vi "Initialize-values.vi"(8 "error in":errorcluster, 11 "UI ref. in":refnum<data-value>) -> (0 "error IO":errorcluster, 3 "UI ref.":refnum<data-value>)   [LabVIEW 2013, in "CameraVision.lvlib" / "CV-UI.lvclass"]
doc: "This function resets the values of the GUI buttons and selectors to consistent defaults.\nThe purpose is to present a consistent GUI after an unexpected program shutdown."
uses:
  CV-UI.lvclass
  CV-UI.lvclass/CV-UI.ctl
  Camera-selector.ctl
  Image-selector.ctl
  Main/Mapping/Mapping-characteristic.ctl
  Settings-source.ctl
  Read Control refs.vi
  Main/Mapping/CV-Mapping.lvclass
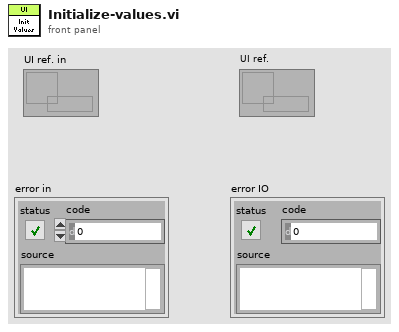
[diagram p1: front panel]
types:
  T1 = typedef "CameraVision.lvlib/CV-UI.lvclass/Camera-selector.ctl" = enum16{"Camera 1", "Camera 2"}
  T2 = typedef "CameraVision.lvlib/CV-UI.lvclass/Image-selector.ctl" = enum16{"Original", "Corrected", "Binary"}
  T3 = typedef "CameraVision.lvlib/CV-Mapping.lvclass/Mapping-characteristic.ctl" = enum16{"Average intensity [0-255]", "Peak intensity [0-255]", "Melt-pool size [mm²]", "Melt-pool aspect ratio []", "Melt-pool fragments []", "Average temperature [°C]", "Max. temperature [°C]", "Min. temperature [°C]", "Std. dev. temperature [°C]"}
  T4 = typedef "CameraVision.lvlib/CV-UI.lvclass/Settings-source.ctl" = enum16{"Custom", "Default", "Last used", "File"}
  T5 = typedef "CameraVision.lvlib/CV-UI.lvclass/Control-names.ctl" = enum16{"Start acquisition", "Activate", "Stop acquisition", "Settings type", "Load settings", "Save settings", "Import images", "Camera selector", "Image type selector", "Batch browser", "Image refresh", "Parameter tabs", "Displays", "Processing tabs", "Processing selector", "Map characteristic", "Show info", "Manual trigger"}
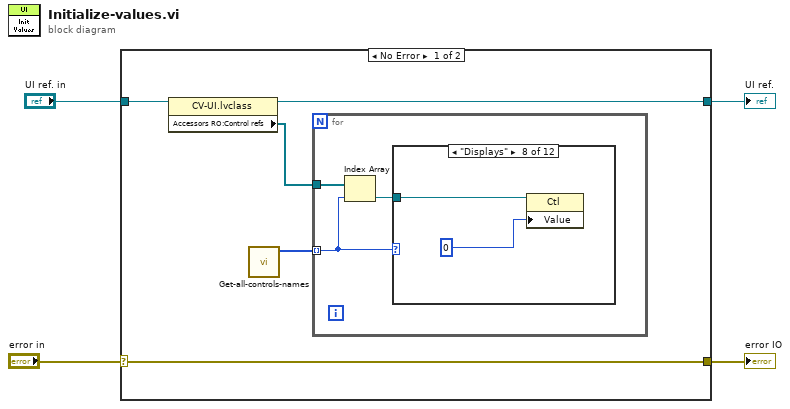
[diagram p0: block diagram]
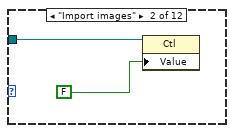
[diagram p3: hidden frame]
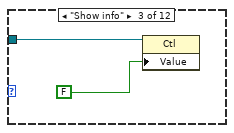
[diagram p4: hidden frame]
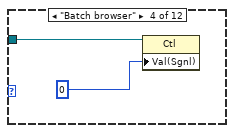
[diagram p5: hidden frame]
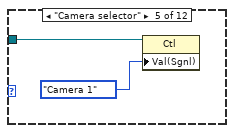
[diagram p6: hidden frame]
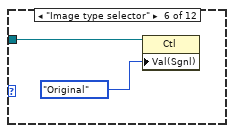
[diagram p7: hidden frame]
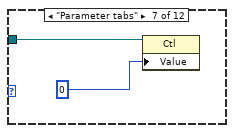
[diagram p8: hidden frame]
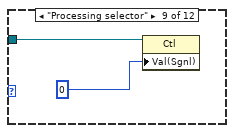
[diagram p9: hidden frame]
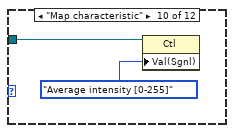
[diagram p10: hidden frame]
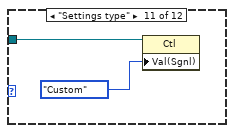
[diagram p11: hidden frame]
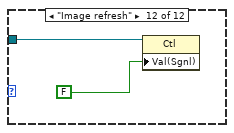
[diagram p12: hidden frame]
diagram:
  n1 = case shown="No Error" "error in" {
    selector: "error in" -> [w5 w36]
    tunnel: "UI ref. in" -> [w7 w35]
    tunnel: [w5 w36] -> w4
    tunnel: [w6 w35] -> w1
    frame No Error {
      n2 = property class="CV-UI.lvclass"(reference=w7) -> (reference out=w6:refnum<data-value>, "Accessors RO:Control refs"=w8:refnum<vi>[])  [unwired: 1 in, 1 out]
      n3 = call "Get-all-controls-names.vi"() -> ("Controls"=w9:T5[])  [unwired: 11 in]
      n4 = for {
        tunnel: w9 -> [w10] mode=indexing
        tunnel: w8 -> [w12]
        n5 = Index Array(array=w12, index=w10) -> (element=w11:refnum<vi>)
        n6 = case shown="\"Displays\"" w10 {
          tunnel: w11 -> [_ w14 w16 w18 w20 w22 w24 w26 w28 w30 w32 w34]
          frame Default {
          }
          frame "Import images" {
            n7 = property class="Ctl"(reference=w14, "Value"=FALSE) -> ()  [unwired: 1 in, 2 out]
          }
          frame "Show info" {
            n8 = property class="Ctl"(reference=w16, "Value"=FALSE) -> ()  [unwired: 1 in, 2 out]
          }
          frame "Batch browser" {
            n9 = property class="Ctl"(reference=w18, "Val(Sgnl)"=0) -> ()  [unwired: 1 in, 2 out]
          }
          frame "Camera selector" {
            n10 = property class="Ctl"(reference=w20, "Val(Sgnl)"=Camera-selector."Camera 1" ("Value")) -> ()  [unwired: 1 in, 2 out]
          }
          frame "Image type selector" {
            n11 = property class="Ctl"(reference=w22, "Val(Sgnl)"=Image-selector."Original" ("Value")) -> ()  [unwired: 1 in, 2 out]
          }
          frame "Parameter tabs" {
            n12 = property class="Ctl"(reference=w24, "Value"=0) -> ()  [unwired: 1 in, 2 out]
          }
          frame "Displays" {
            n13 = property class="Ctl"(reference=w26, "Value"=0) -> ()  [unwired: 1 in, 2 out]
          }
          frame "Processing selector" {
            n14 = property class="Ctl"(reference=w28, "Val(Sgnl)"=0) -> ()  [unwired: 1 in, 2 out]
          }
          frame "Map characteristic" {
            n15 = property class="Ctl"(reference=w30, "Val(Sgnl)"=Mapping-characteristic."Average intensity [0-255]" ("Value")) -> ()  [unwired: 1 in, 2 out]
          }
          frame "Settings type" {
            n16 = property class="Ctl"(reference=w32, "Val(Sgnl)"=Settings-source."Custom" ("Value (Signaling)")) -> ()  [unwired: 1 in, 2 out]
          }
          frame "Image refresh" {
            n17 = property class="Ctl"(reference=w34, "Val(Sgnl)"=FALSE) -> ()  [unwired: 1 in, 2 out]
          }
        }
      }
    }
    frame Error {
    }
  }
  "error IO" <- w4
  "UI ref." <- w1
